vi "Blocks.vi"(1 "Input Picture":picture, 2 "Width":i16=30, 3 "Origin Y":i16, 4 "Origin X":i16) -> (0 "?":picture)   [LabVIEW 2014]
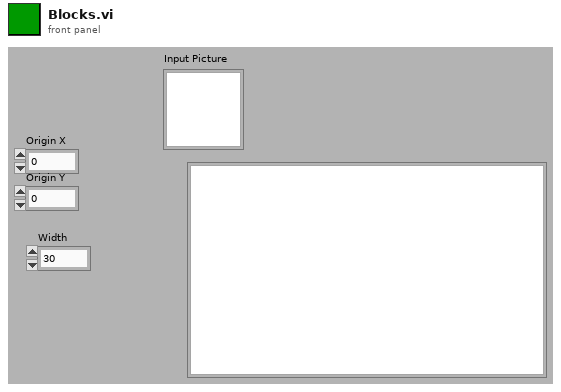
[diagram p1: front panel]
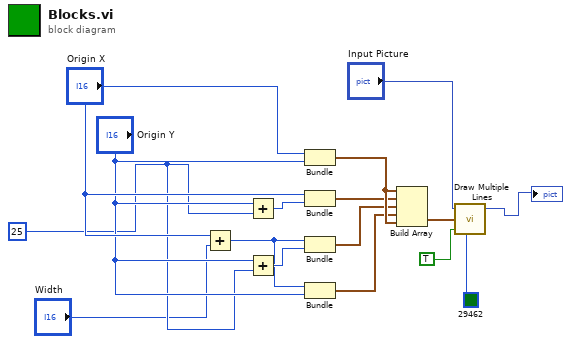
[diagram p0: block diagram]
diagram:
  w3 = i16 25 ("Height")
  n1 = Add(x="Origin X", y="Width") -> (x+y=w9:i16)
  n2 = Add(x="Origin Y", y=w3) -> (x+y=w12:i16)
  n3 = Add(x="Origin Y", y=w3) -> (x+y=w10:i16)
  n4 = Bundle("Origin X"="Origin X", "Origin Y"="Origin Y") -> (w16:cluster{"Origin X":i16, "Origin Y":i16})  [unwired: 1 in]
  n5 = Bundle("Origin X"="Origin X", w12) -> (w14:cluster{"Origin X":i16, i16})  [unwired: 1 in]
  n6 = Bundle(w9, w10) -> (w11:cluster{i16, i16})  [unwired: 1 in]
  n7 = Bundle(w9, "Origin Y"="Origin Y") -> (w7:cluster{i16, "Origin Y":i16})  [unwired: 1 in]
  n8 = Build Array(w16, w14, w11, w7, w16) -> (w15:cluster{"Origin X":i16, "Origin Y":i16}[])
  n9 = call <vilib>:"Draw Multiple Lines.vi"("picture"="Input Picture", "line endpoints"=w15, "fill?(F)"=TRUE, "color(black)"=u32 29462) -> ("new picture"=→"?":picture)  [unwired: 5 in]
